vi "Space Deletion.vi"(1 "string with spaces":string) -> (0 "string without spaces":string)   [LabVIEW 2010, in "NI_Gmath.lvlib"]
uses:
  NI_Gmath.lvlib
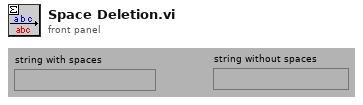
[diagram p1: front panel]
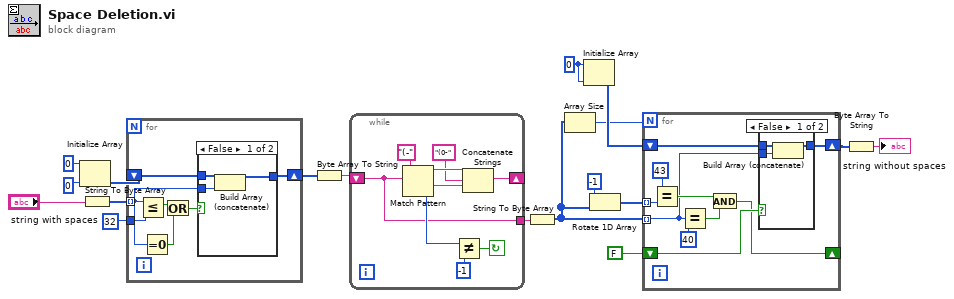
[diagram p0: block diagram]
diagram:
  w6 = 0
  n1 = Initialize Array(u8 0, 0) -> (w15:u8[])
  n2 = String To Byte Array(string="string with spaces") -> (unsigned byte array=w11:u8[])
  n3 = for {
    shift-right: [w23] -> w13
    shift-left: w15 -> [w24]
    tunnel: w11 -> [w22] mode=indexing
    tunnel: u8 32 -> [w25]
    n4 = Less Or Equal?(x=w22, y=w25) -> (x <= y?=w20:bool)
    n5 = Equal To 0?(x=w22) -> (x = 0?=w21:bool)
    n6 = Or(x=w20, y=w21) -> (x .or. y?=w19:bool)
    n7 = case shown="False" w19 {
      tunnel: w24 -> [w28 w29]
      tunnel: [w27 w29] -> w23
      tunnel: w22 -> [w26 _]
      frame False {
        n8 = Build Array (concatenate)(w28, w26) -> (w27:u8[])
      }
      frame True {
      }
    }
  }
  n9 = Byte Array To String(unsigned byte array=w13) -> (string=w12:string)
  n10 = while {
    tunnel: [w30] -> w8
    shift-left: w12 -> [w30]
    shift-right: [w34] -> _
    stop <- w31 continue-if-true
    n11 = Match Pattern(string=w30, regular expression="(-") -> (before substring=w37:string, after substring=w35:string, offset past match=w33:i32)  [unwired: 1 in, 1 out]
    n12 = Not Equal?(x=w33, y=-1) -> (x != y?=w31:bool)
    n13 = Concatenate Strings(w37, "(0-", w35) -> (w34:string)
  }
  n14 = String To Byte Array(string=w8) -> (unsigned byte array=w4:u8[])
  n15 = Array Size(array=w4) -> (size(s)=w1:i32)
  n16 = Initialize Array(w6, w6) -> (w5:i32[])
  n17 = Rotate 1D Array(1:w4, 2:-1) -> (0:w3:u8[])
  n18 = for {
    N: w1 -> [_]
    tunnel: w3 -> [w48] mode=indexing
    tunnel: w4 -> [w41] mode=indexing
    shift-right: [w42] -> w9
    shift-left: w5 -> [w43]
    shift-right: [w39] -> _
    shift-left: FALSE -> [w40]
    n19 = Equal?(x=43, y=w48) -> (x = y?=w45:bool)
    n20 = Equal?(x=w41, y=40) -> (x = y?=w44:bool)
    n21 = And(x=w45, y=w44) -> (x .and. y?=w39:bool)
    n22 = case shown="False" w40 {
      tunnel: w43 -> [w51 w52]
      tunnel: [w50 w52] -> w42
      tunnel: w41 -> [w49 _]
      frame False {
        n23 = Build Array (concatenate)(w51, w49) -> (w50:i32[])
      }
      frame True {
      }
    }
  }
  n24 = Byte Array To String(unsigned byte array=w9) -> (string=→"string without spaces":string)
